vi "EnableDisable.vi"(7 "ch":i32, 8 "error in (no error)":errorcluster, 10 "Enable":bool, 11 "MagiQmw3 in":refnum<class "MagiQmw3.lvclass">) -> (0 "error out":errorcluster, 3 "MagiQmw3 out":refnum<class "MagiQmw3.lvclass">)   [LabVIEW 2012, in "MagiQmw3.lvclass"]
uses:
  MagiQmw3.lvclass
  MagiQmw3.lvclass/MagiQmw3.ctl
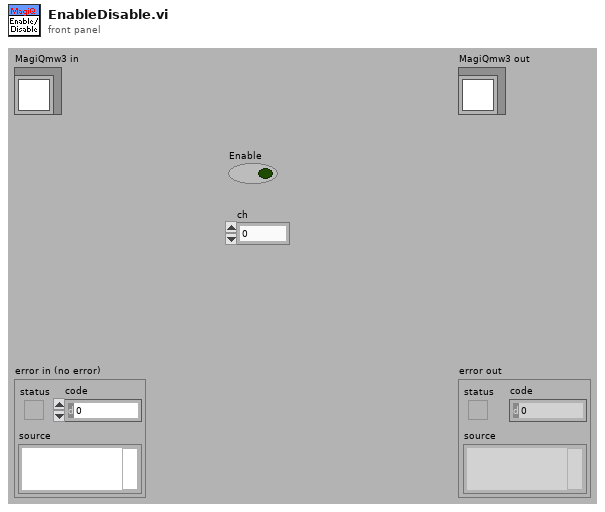
[diagram p1: front panel]
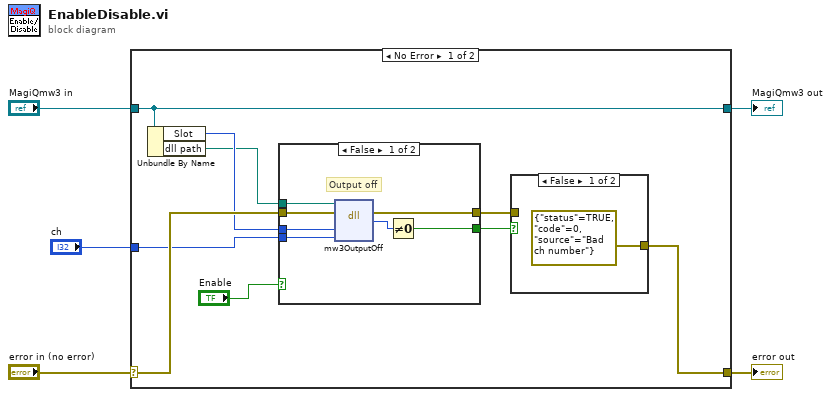
[diagram p0: block diagram]
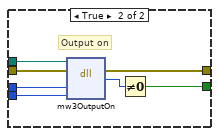
[diagram p3: hidden frame]
diagram:
  n1 = case shown="No Error" "error in (no error)" {
    selector: "error in (no error)" -> [w13 w32]
    tunnel: [w7 w32] -> w4
    tunnel: [w14 w31] -> w2
    tunnel: "MagiQmw3 in" -> [w14 w31]
    tunnel: "ch" -> [w11 _]
    frame No Error {
      n2 = Unbundle By Name(w14) -> ("Slot"=w12:u16, "dll path"=w6:path)
      n3 = case shown="False" "Enable" {
        tunnel: w13 -> [w22 w30]
        tunnel: [w21 w29] -> w8
        tunnel: w12 -> [w20 w28]
        tunnel: w11 -> [w19 w27]
        tunnel: [w18 w25] -> w9
        tunnel: w6 -> [w17 w24]
        frame False {
          # "Output off"
          n4 = dll-call lib="PulserLib.dll" fn="mw3OutputOff"(path in=w17, error in=w22, "slot"=w20, "ch"=w19) -> (error out=w21:errorcluster, "return"=w23:i32)  [unwired: 3 in, 1 out]
          n5 = Not Equal To 0?(x=w23) -> (x != 0?=w18:bool)
        }
        frame True {
          # "Output on"
          n6 = dll-call lib="PulserLib.dll" fn="mw3OutputOn"(path in=w24, error in=w30, "slot"=w28, "ch"=w27) -> (error out=w29:errorcluster, "return"=w26:i32)  [unwired: 3 in, 1 out]
          n7 = Not Equal To 0?(x=w26) -> (x != 0?=w25:bool)
        }
      }
      n8 = case shown="False" w9 {
        tunnel: w8 -> [_ w16]
        tunnel: [errorcluster {"status"=TRUE, "code"=0, "source"="Bad ch number"} ("error in (no error)") w16] -> w7
        frame False {
        }
        frame True {
        }
      }
    }
    frame Error {
    }
  }
  "error out" <- w4
  "MagiQmw3 out" <- w2
